vi "Z6_Beamline.Calc Frontends State.vi"(0 "i ref in":refnum<vi>, 5 "error in (no error)":errorcluster) -> (14 "i ref out":refnum<vi>, 19 "error out":errorcluster)   [LabVIEW 2014, in "Z6_Beamline.lvlib"]
doc: "This VI calculates the Frontends state of the Z6 Beamline."
uses:
  Z6_Beamline.lvlib
  PH_Common/PH_Common.lvlib
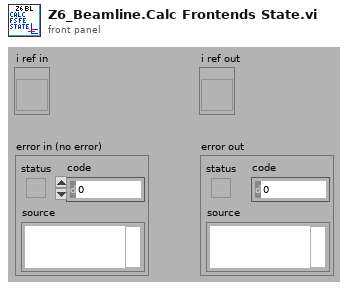
[diagram p1: front panel]
types:
  T1 = typedef "Z6_Beamline.lvlib/Z6_Beamline.i attribute.ctl" = cluster{"Subs ok GUI Refs":T2, "Refs BL Northtower":refnum<vi>[], "Refs BL Southtower":refnum<vi>[], "Refs BL 100TW COS":refnum<vi>[], "State Subsystems":cluster{"Northtower":bool, "Southtower":bool, "Frontends":bool, "100TW COS":bool}, "Z6 Beamline Status Subscriber Information":T3, "Color State PHELIX":i16}
  T2 = typedef "Z6_Beamline.lvlib/Z6_Beamline.Subsystem ok GUI Refs.ctl" = cluster{"Northtower ok":refnum<vi>, "Southtower ok":refnum<vi>, "Frontends ok":refnum<vi>, "100TW COS ok":refnum<vi>}
  T3 = typedef "Z6_Beamline.lvlib/Z6_Beamline.Status Subscriber Information.ctl" = cluster{"BL Z6 Shutter":T4, "CH 10":T4, "CH 11":T4, "ST Flip Cam":T4, "ST Flip DB":T4, "BL Z6 Dump":T4}
  T4 = typedef "PH_BL-Master.lvlib/PH_BL-Master.Status Subscriber Information.ctl" = cluster{"Index of element":i32, "Attributeset":T5}
  T5 = typedef "PH_BL-Master.lvlib/PH_BL-Master.Attribute Set.ctl" = enum16{"Boolean Status Service Subscriber", "Picture Status Service Subscriber"}
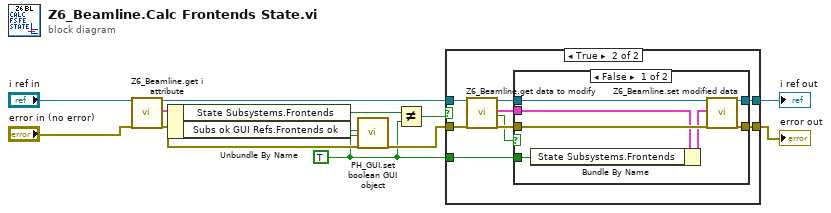
[diagram p0: block diagram]
diagram:
  w1 = TRUE ("Northtower R2S")
  n1 = call "Z6_Beamline.get i attribute.vi"("i ref in"="i ref in", "error in (no error)"="error in (no error)") -> ("i ref out"=w7:refnum<vi>, "i attribute"=w12:T1, "error out"=w10:errorcluster)  [unwired: 15 in]
  n2 = Unbundle By Name(w12) -> ("State Subsystems.Frontends"=w2:bool, "Subs ok GUI Refs.Frontends ok"=w11:refnum<vi>)
  n3 = call "PH_GUI.set boolean GUI object.vi"("Boolean Knob GUI Ref"=w11, "Value"=w1, "error in (no error)"=w10) -> ("error out"=w5:errorcluster)  [unwired: 16 in]
  n4 = Not Equal?(x=w2, y=w1) -> (x != y?=w3:bool)
  n5 = case shown="True" w3 {
    tunnel: w7 -> [w14 w19]
    tunnel: [w14 w18] -> w6
    tunnel: w5 -> [w13 w17]
    tunnel: [w13 w16] -> w4
    tunnel: w1 -> [_ w15]
    frame False {
    }
    frame True {
      n6 = call "Z6_Beamline.get data to modify.vi"("i ref in"=w19, "error in (no error)"=w17) -> ("i ref out"=w22:refnum<vi>, "i attribute"=w20:T1, "timed out"=w21:bool, "error out"=w23:errorcluster)  [unwired: 14 in]
      n7 = case shown="False" w21 {
        tunnel: w23 -> [w30 w31]
        tunnel: w22 -> [w29 w32]
        tunnel: [w28 w31] -> w16
        tunnel: [w27 w32] -> w18
        tunnel: w20 -> [w26 _]
        tunnel: w15 -> [w24 _]
        frame False {
          n8 = Bundle By Name(cluster=w26, "State Subsystems.Frontends"=w24) -> (w25:T1)
          n9 = call "Z6_Beamline.set modified data.vi"("i ref in"=w29, "i attribute"=w25, "error in (no error)"=w30) -> ("i ref out"=w27:refnum<vi>, "error out"=w28:errorcluster)  [unwired: 15 in]
        }
        frame True {
        }
      }
    }
  }
  "i ref out" <- w6
  "error out" <- w4
